vi "Check_Elevator.vi"(8 "error in (no error)":errorcluster, 11 "Elevator in":T1) -> (0 "error out":errorcluster, 2 "Open Doors?":bool, 3 "Elevator out":T1)   [LabVIEW 2026]
uses:
  Controls/Elevator_Status.ctl
  Controls/Door_Status_Enum.ctl
  Controls/Occupy_Status.ctl
  Controls/Floor_Status.ctl
  Controls/Motion_Status_Enum.ctl
  Controls/Car_Calls_Status.ctl
  Controls/Hall_Calls_Status.ctl
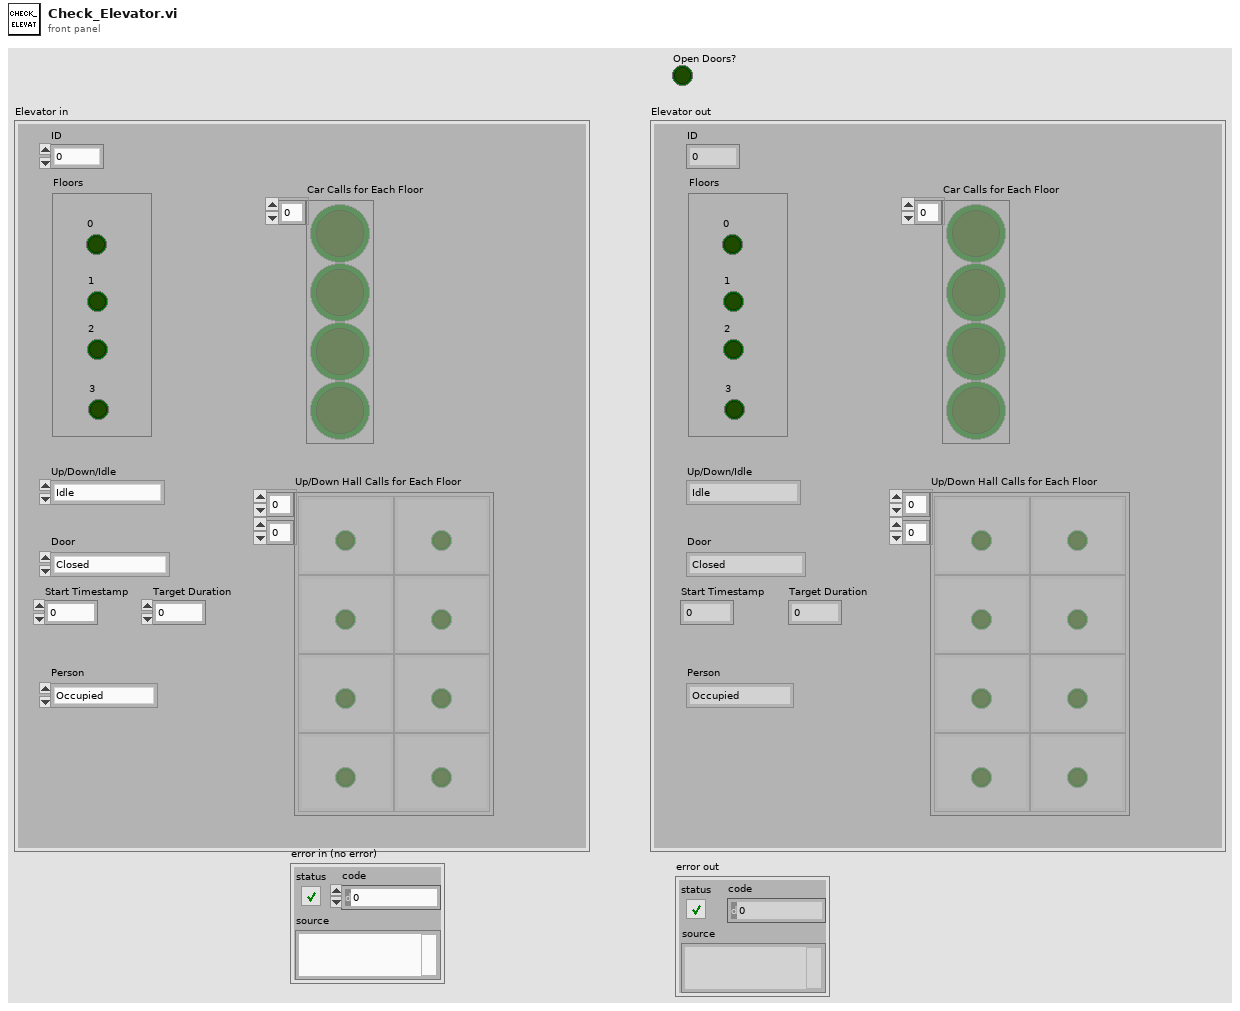
[diagram p1: front panel]
types:
  T1 = typedef "Elevator_Status.ctl" = cluster{"Door":T2, "Person":T3, "Floors":T4, "Up/Down/Idle":T5, "Car Calls for Each Floor":T6, "Up/Down Hall Calls for Each Floor":T7, "ID":i32, "Start Timestamp":u32, "Target Duration":dbl}
  T2 = typedef "Door_Status_Enum.ctl" = enum16{"Closed", "Open", "Opening", "Closing"}
  T3 = typedef "Occupy_Status.ctl" = enum16{"Occupied", "Empty"}
  T4 = typedef "Floor_Status.ctl" = cluster{"0":bool, "1":bool, "2":bool, "3":bool}
  T5 = typedef "Motion_Status_Enum.ctl" = enum16{"Idle", "Up", "Down"}
  T6 = typedef "Car_Calls_Status.ctl" = bool[]
  T7 = typedef "Hall_Calls_Status.ctl" = cluster{bool}[][]
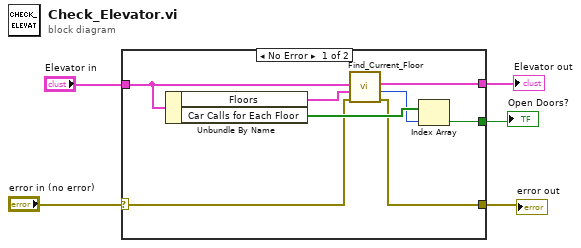
[diagram p0: block diagram]
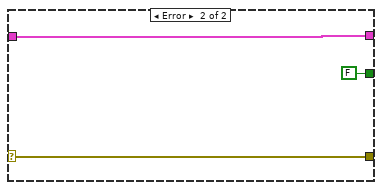
[diagram p2: hidden frame]
diagram:
  n1 = case shown="No Error" "error in (no error)" {
    selector: "error in (no error)" -> [w10 w16]
    tunnel: [w12 FALSE ("Boolean")] -> w5
    tunnel: "Elevator in" -> [w6 w14]
    tunnel: [w9 w16] -> w2
    tunnel: [w8 w14] -> w1
    frame No Error {
      n2 = Unbundle By Name(w6) -> ("Floors"=w7:T4, "Car Calls for Each Floor"=w13:T6)
      n3 = call "Find_Current_Floor.vi"("error in (no error)"=w10, "Floors"=w7, "Elevator Status in"=w6) -> ("error out"=w9:errorcluster, "Current Floor"=w11:i32, "Elevator Status out"=w8:T1)  [unwired: 5 in, 1 out]
      n4 = Index Array(array=w13, index=w11) -> (element=w12:bool)
    }
    frame Error {
    }
  }
  "Open Doors?" <- w5
  "Elevator out" <- w1
  "error out" <- w2
